vi "set_x.vi"(8 "error in":errorcluster, 11 "x_value_um":dbl format="%0.2f") -> (0 "error out":errorcluster)   [LabVIEW 2018]
uses:
  <vilib>/DAQmx/write.llb/DAQmx Write (Analog DBL 1Chan 1Samp).vi
  GLOBAL_VAR.vi
  <vilib>/DAQmx/create/channels.llb/DAQmx Create Channel (AO-Voltage-Basic).vi
  <vilib>/DAQmx/miscellaneous.llb/DAQmx Fill In Error Info.vi
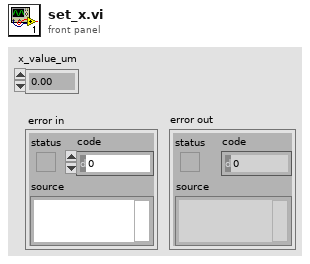
[diagram p1: front panel]
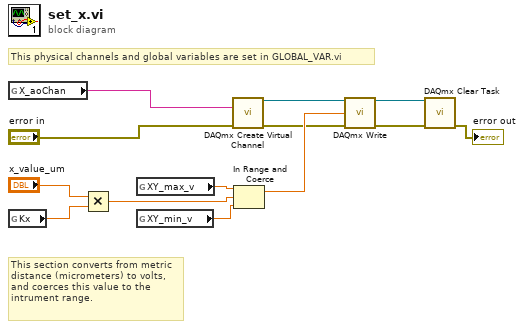
[diagram p0: block diagram]
diagram:
  # "This physical channels and global variables are set in GLOBAL_VAR.vi"
  # "This section converts from metric distance (micrometers) to volts, and coerces this value to the intrument range."
  n1 = global read "GLOBAL_VAR.vi" "X_aoChan"() -> (w11:tag)
  n2 = global read "GLOBAL_VAR.vi" "Kx"() -> (w4:dbl)
  n3 = Multiply(x="x_value_um", y=w4) -> (x*y=w1:dbl)
  n4 = global read "GLOBAL_VAR.vi" "XY_max_v"() -> (w3:dbl)
  n5 = global read "GLOBAL_VAR.vi" "XY_min_v"() -> (w2:dbl)
  n6 = call-poly <vilib>:"DAQmx Create Virtual Channel.vi"("physical channels"=w11, "error in"="error in") -> ("task out"=w12:refnum<k21>, "error out"=w8:errorcluster)  [unwired: 12 in]
  n7 = In Range and Coerce(upper limit=w3, x=w1, lower limit=w2) -> (coerced(x)=w10:dbl)  [unwired: 1 out]
  n8 = call-poly <vilib>:"DAQmx Write.vi"("task/channels in"=w12, "data"=w10, "error in"=w8) -> ("task out"=w13:refnum<k21>, "error out"=w7:errorcluster)  [unwired: 10 in, 1 out]
  n9 = call <vilib>:"DAQmx Clear Task.vi"("task in"=w13, "error in"=w7) -> ("error out"=→"error out":errorcluster)  [unwired: 13 in]
